vi "Ch_data_pattern_16_save (SubVI).vi"(7 "error in":errorcluster, 10 "R1-8 Cluster":T1, 11 "P S1":dbl, 12 "T1-2 Cluster":cluster{"T1":dbl, "T2":dbl}, 13 "P S2":dbl, 15 "Activate!":bool, 17 "file":refnum<file>) -> (27 "error out":errorcluster)   [LabVIEW 2015]
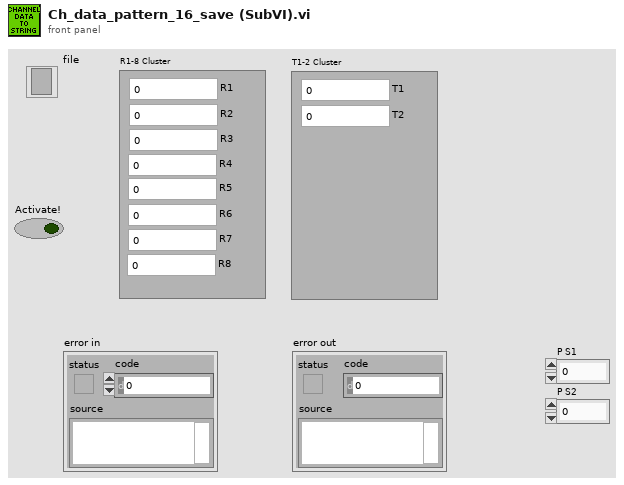
[diagram p1: front panel]
types:
  T1 = cluster{"R1":dbl, "R2":dbl, "R3":dbl, "R4":dbl, "R5":dbl, "R6":dbl, "R7":dbl, "R8":dbl}
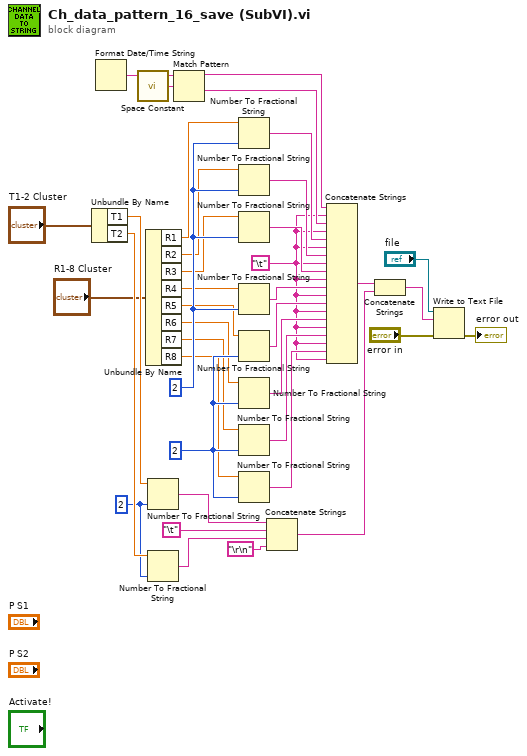
[diagram p0: block diagram]
diagram:
  w8 = i16 2 ("precision (6)")
  w27 = i16 2 ("precision (6)")
  w37 = i16 2 ("precision (6)")
  w14 = "\t"
  n1 = Unbundle By Name("T1-2 Cluster") -> ("T1"=w10:dbl, "T2"=w11:dbl)
  n2 = Format Date/Time String() -> (date/time string=w29:string)  [unwired: 3 out]
  n3 = call <vilib>:"Space Constant.vi"() -> ("String"=w30:string)
  n4 = Unbundle By Name("R1-8 Cluster") -> ("R1"=w22:dbl, "R2"=w21:dbl, "R3"=w20:dbl, "R4"=w19:dbl, "R5"=w18:dbl, "R6"=w17:dbl, "R7"=w16:dbl, "R8"=w15:dbl)
  n5 = Number To Fractional String(number=w10, precision (6)=w8) -> (F-format string=w9:string)  [unwired: 2 out]
  n6 = Number To Fractional String(number=w11, precision (6)=w8) -> (F-format string=w5:string)  [unwired: 2 out]
  n7 = Match Pattern(string=w29, regular expression=w30) -> (before substring=w31:string, after substring=w32:string)  [unwired: 3 out]
  n8 = Number To Fractional String(number=w22, precision (6)=w37) -> (F-format string=w33:string)  [unwired: 2 out]
  n9 = Number To Fractional String(number=w21, precision (6)=w37) -> (F-format string=w34:string)  [unwired: 2 out]
  n10 = Number To Fractional String(number=w20, precision (6)=w37) -> (F-format string=w35:string)  [unwired: 2 out]
  n11 = Number To Fractional String(number=w19, precision (6)=w37) -> (F-format string=w36:string)  [unwired: 2 out]
  n12 = Number To Fractional String(number=w18, precision (6)=w27) -> (F-format string=w26:string)  [unwired: 2 out]
  n13 = Number To Fractional String(number=w17, precision (6)=w27) -> (F-format string=w25:string)  [unwired: 2 out]
  n14 = Number To Fractional String(number=w16, precision (6)=w27) -> (F-format string=w24:string)  [unwired: 2 out]
  n15 = Number To Fractional String(number=w15, precision (6)=w27) -> (F-format string=w23:string)  [unwired: 2 out]
  n16 = Concatenate Strings(w9, "\t", w5, "\r\n") -> (w7:string)
  n17 = Concatenate Strings(w31, w14, w32, w14, w33, w14, w34, w14, w35, w14, w36, w14, w26, w14, w25, w14, w24, w14, w23, w14) -> (w13:string)
  n18 = Concatenate Strings(w13, w7) -> (w12:string)
  n19 = Write to Text File(file (use dialog)="file", text=w12, error in="error in") -> (error out=→"error out":errorcluster)  [unwired: 3 out]
